vi "write N relays.vi"(8 "error in (no error)":errorcluster, 10 "data":bool[](array[boolean])=[TRUE, FALSE, TRUE, FALSE], 11 "Relays in":refnum<class "Relays.lvclass">) -> (0 "error out":errorcluster, 3 "Relays out":refnum<class "Relays.lvclass">)   [LabVIEW 2025, in "Relays.lvclass"]
uses:
  Relays.lvclass
  Relays.lvclass/Relays.ctl
  <vilib>/DAQmx/write.llb/DAQmx Write (Digital 1D Bool NChan 1Samp 1Line).vi
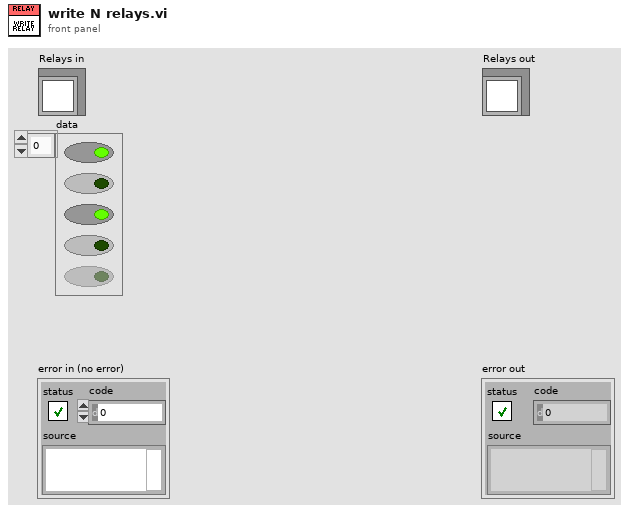
[diagram p1: front panel]
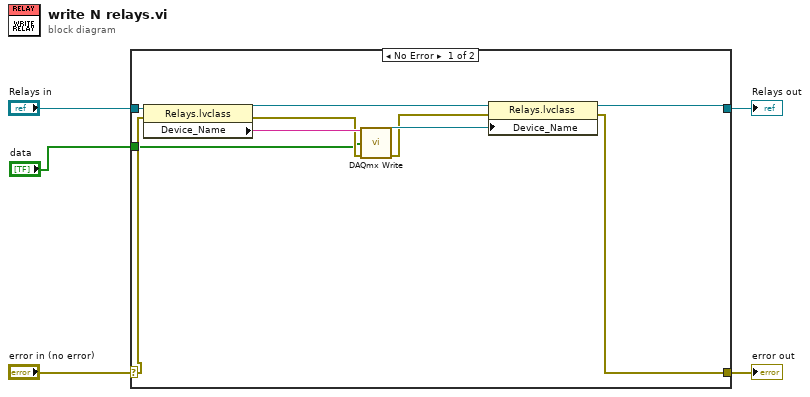
[diagram p0: block diagram]
diagram:
  n1 = case shown="No Error" "error in (no error)" {
    selector: "error in (no error)" -> [w14 w17]
    tunnel: [w7 w17] -> w4
    tunnel: [w8 w16] -> w2
    tunnel: "Relays in" -> [w15 w16]
    tunnel: "data" -> [w6 _]
    frame No Error {
      n2 = property class="Relays.lvclass"(reference=w15, error in=w14) -> (reference out=w10:refnum<class "Relays.lvclass">, error out=w12:errorcluster, "Device_Name"=w13:string)
      n3 = call-poly <vilib>:"DAQmx Write.vi"("task/channels in"=w13, "data"=w6, "error in"=w12) -> ("task out"=w11:refnum<k21>, "error out"=w9:errorcluster)  [unwired: 10 in, 1 out]
      n4 = property class="Relays.lvclass"(reference=w10, error in=w9, "Device_Name"=w11) -> (reference out=w8:refnum<class "Relays.lvclass">, error out=w7:errorcluster)
    }
    frame Error {
    }
  }
  "error out" <- w4
  "Relays out" <- w2
